vi "Global_tst_num.vi"() -> ()   [LabVIEW 2020]
panel:
  in  "num":dbl format="%.2f"
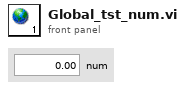
[diagram p1: front panel]
diagram:
